vi "Semaphore Size.vi"(8 "error in (no error)":errorcluster, 11 "Semaphore in":T1) -> (0 "error out":errorcluster, 2 "sem_t size (bytes)":u64, 3 "Semaphore out":T1)   [LabVIEW 2013, in "POSIX Threads.lvlib" / "Semaphore.lvclass"]
doc: "Returns the size of a pthread sempahore object in memory."
uses:
  Semaphore.lvclass
  Controls/reference.ctl
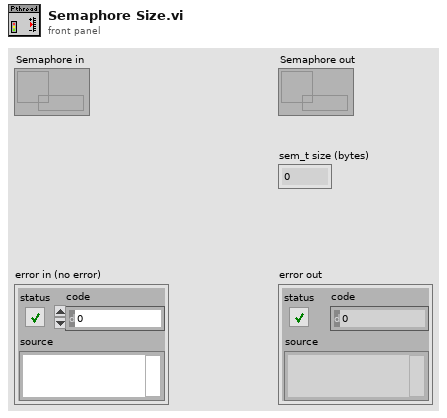
[diagram p1: front panel]
types:
  T1 = typedef "POSIX Threads.lvlib/Semaphore.lvclass/reference.ctl" = refnum<data-value>
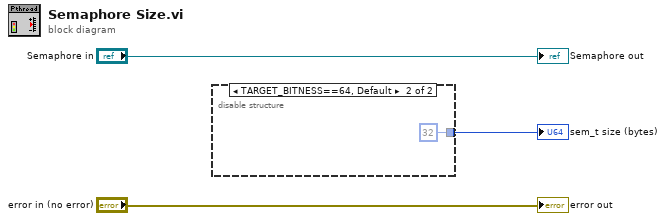
[diagram p0: block diagram]
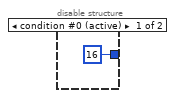
[diagram p2: hidden frame]
diagram:
  n1 = disable-structure shown="TARGET_BITNESS==64, Default" {
    disable-tunnel: [u64 16 ("sem_t size (bytes)") u64 32 ("sem_t size (bytes)")] -> w1
    frame condition #0 (active) {
    }
    frame condition #1 {
    }
  }
  "sem_t size (bytes)" <- w1
  "error out" <- "error in (no error)"
  "Semaphore out" <- "Semaphore in"
